vi "Actualiza Credito.vi"(8 "error in (no error)":errorcluster, 10 "CREDITO ACTUAL":dbl, 11 "UI Actor in":refnum<class "UI Actor.lvclass">) -> (0 "error out":errorcluster, 3 "UI Actor out":refnum<class "UI Actor.lvclass">)   [LabVIEW 2019, in "UI Actor.lvlib" / "UI Actor.lvclass"]
uses:
  UI Actor.lvclass
  UI Actor.lvclass/UI Actor.ctl
  MENSAJES Messages/Actualiza Mensaje Msg/Actualiza Mensaje Msg.lvclass/Actualiza Mensaje Msg.ctl
  <vilib>/ActorFramework/Message Enqueuer/Message Enqueuer.lvclass/Message Enqueuer.ctl
  <vilib>/ActorFramework/Message Enqueuer/Enqueue.vi
  MENSAJES Messages/Actualiza Mensaje Msg/Actualiza Mensaje Msg.lvclass
  C:/Program Files (x86)/National Instruments/LabVIEW 2019/vi.lib/ActorFramework/Message/Message.lvclass
  <vilib>/ActorFramework/Message Priority Queue/Priority Enqueue.vi
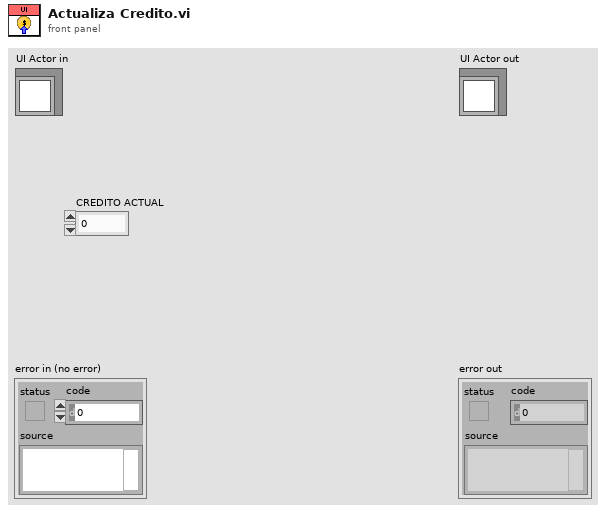
[diagram p1: front panel]
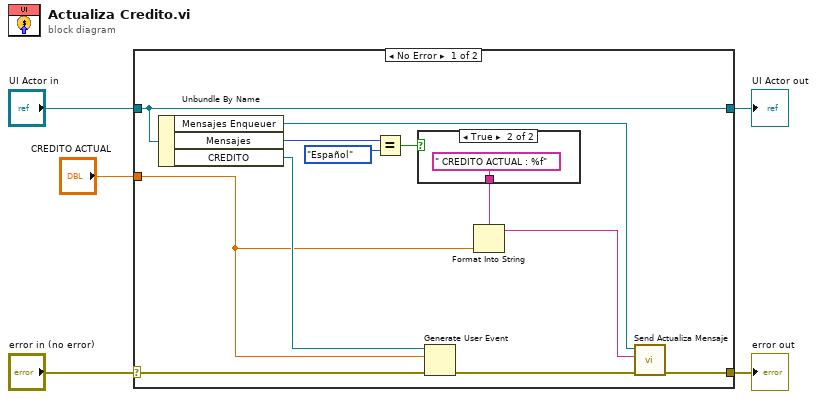
[diagram p0: block diagram]
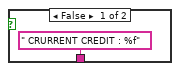
[diagram p2: hidden frame]
diagram:
  n1 = case shown="No Error" "error in (no error)" {
    selector: "error in (no error)" -> [w17 w21]
    tunnel: [w13 w21] -> w4
    tunnel: [w16 w20] -> w2
    tunnel: "UI Actor in" -> [w16 w20]
    tunnel: "CREDITO ACTUAL" -> [w12 _]
    frame No Error {
      n2 = Unbundle By Name(w16) -> ("Mensajes Enqueuer"=w9:refnum<class "Message Enqueuer.lvclass">, "Mensajes"=w8:enum16{"Ingles", "Español"}, "CREDITO"=w15:refnum<user-event>)
      n3 = Equal?(x=w8, y=enum16{"Ingles", "Español"}."Español") -> (x = y?=w6:bool)
      n4 = case shown="True" w6 {
        tunnel: [" CRURRENT CREDIT : %f" ("format string") " CREDITO ACTUAL : %f" ("format string")] -> w10
        frame False {
        }
        frame True {
        }
      }
      n5 = Generate User Event(user event=w15, event data cluster=w12, error in=w17) -> (error out=w14:errorcluster)  [unwired: 1 in, 1 out]
      n6 = Format Into String(format string=w10, w12) -> (resulting string=w11:string)  [unwired: 2 in, 1 out]
      n7 = call "Send Actualiza Mensaje.vi"("error in (no error)"=w14, "Mensaje Status"=w11, "Message Enqueuer"=w9) -> ("error out"=w13:errorcluster)  [unwired: 7 in, 1 out]
    }
    frame Error {
    }
  }
  "error out" <- w4
  "UI Actor out" <- w2
